vi "dfd_Group Delay_Integer Tau.vi"(7 "parameter":cluster{"epsilon":dbl, "times":i32}={"epsilon"=0.0001, "times"=200}, 8 "error in (no error)":errorcluster, 10 "Coefficients (in)":cluster{"r":dbl[], "theta":dbl[], "offset":dbl}, 11 "Design Info":T1={"p"=2, "freq grid"=[], "d"=[], "weight"=[], "Order"=0, "radius"=1.0}) -> (0 "error out":errorcluster, 1 "Error":dbl, 2 "Coefficients (out)":cluster{"r":dbl[], "theta":dbl[], "offset":dbl})   [LabVIEW 2017, in "NI_DigFilter_Design.lvlib"]
uses:
  <vilib>/addons/Digital Filter Design/NI_DigFilter_Design.lvlib
  <vilib>/addons/Digital Filter Design/_GroupDelay.llb/dfd_Group Delay_Design Info.ctl
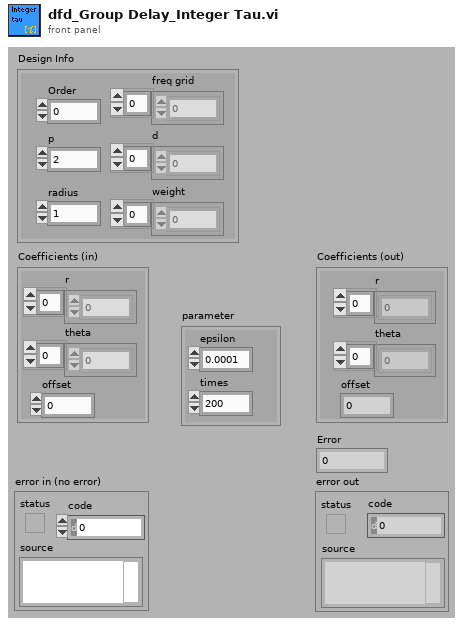
[diagram p1: front panel]
types:
  T1 = typedef "dfd_Group Delay_Design Info.ctl" = cluster{"p":i32, "freq grid":dbl[], "d":dbl[], "weight":dbl[], "Order":i32, "radius":dbl}
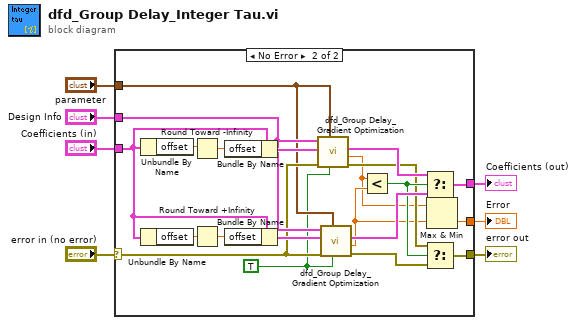
[diagram p0: block diagram]
diagram:
  n1 = case shown="No Error" "error in (no error)" {
    selector: "error in (no error)" -> [w8 w22]
    tunnel: "Design Info" -> [_ w23]
    tunnel: "Coefficients (in)" -> [_ w20]
    tunnel: "parameter" -> [_ w21]
    tunnel: [_ w11] -> w1
    tunnel: [_ w10] -> w4
    tunnel: [w8 w9] -> w3
    frame Error {
    }
    frame No Error {
      w19 = TRUE ("integer tau")
      n2 = Unbundle By Name(w20) -> ("offset"=w27:dbl)
      n3 = Unbundle By Name(w20) -> ("offset"=w28:dbl)
      n4 = Round Toward -Infinity(1:w27) -> (0:w26:dbl)
      n5 = Round Toward +Infinity(x=w28) -> (ceil(x): smallest int >= x=w29:dbl)
      n6 = Bundle By Name(cluster=w20, "offset"=w26) -> (w25:cluster{"r":dbl[], "theta":dbl[], "offset":dbl})
      n7 = Bundle By Name(cluster=w20, "offset"=w29) -> (w24:cluster{"r":dbl[], "theta":dbl[], "offset":dbl})
      n8 = call <vilib>:"dfd_Group Delay_Gradient Optimization.vi"("modify offset"=w19, "parameter"=w21, "error in (no error)"=w22, "Coefficients (in)"=w25, "Design Info"=w23) -> ("error out"=w15:errorcluster, "Error"=w12:dbl, "Coefficients (out)"=w18:cluster{"r":dbl[], "theta":dbl[], "offset":dbl})  [unwired: 4 out]
      n9 = call <vilib>:"dfd_Group Delay_Gradient Optimization.vi"("modify offset"=w19, "parameter"=w21, "error in (no error)"=w22, "Coefficients (in)"=w24, "Design Info"=w23) -> ("error out"=w14:errorcluster, "Error"=w13:dbl, "Coefficients (out)"=w17:cluster{"r":dbl[], "theta":dbl[], "offset":dbl})  [unwired: 4 out]
      n10 = Less?(x=w12, y=w13) -> (x < y?=w16:bool)
      n11 = Select(t=w18, s=w16, f=w17) -> (s? t:f=w11:cluster{"r":dbl[], "theta":dbl[], "offset":dbl})
      n12 = Select(t=w15, s=w16, f=w14) -> (s? t:f=w9:errorcluster)
      n13 = Max & Min(x=w12, y=w13) -> (min(x,y)=w10:dbl)  [unwired: 1 out]
    }
  }
  "Error" <- w4
  "error out" <- w3
  "Coefficients (out)" <- w1
